vi "Config-Stress-Definition.vi"(6 "delete all units":bool, 8 "error in (no error)":errorcluster, 9 "comments (max 58 chars)":string, 10 "trigger (disable:0)":u16(ring), 11 "VISA session":refnum<visa-resource-name>) -> (0 "error out":errorcluster, 3 "VISA resource name out":refnum<visa-resource-name>)   [LabVIEW 2016, in "Agilent 415X Series.lvlib"]
doc: "This VI configures stress setting shared by all units (on stress group level)."
uses:
  Agilent 415X Series.lvlib
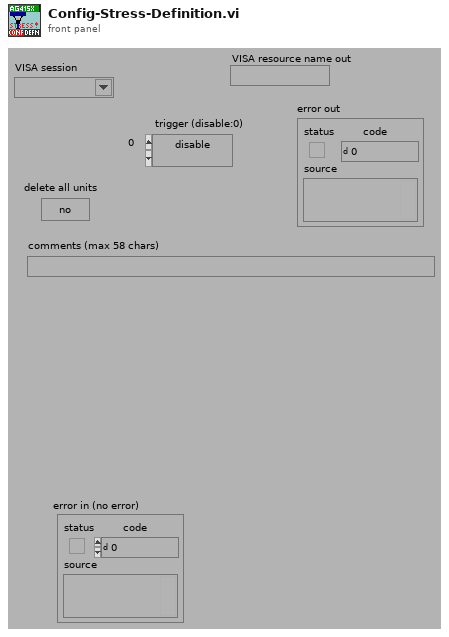
[diagram p1: front panel]
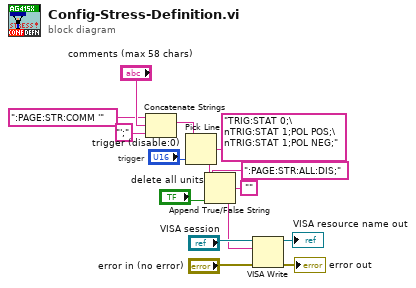
[diagram p0: block diagram]
diagram:
  # "trigger"
  n1 = Concatenate Strings(":PAGE:STR:COMM '", "comments (max 58 chars)", "';") -> (w11:string)
  n2 = Pick Line(string ("")=w11, multi-line string="TRIG:STAT 0;\nTRIG:STAT 1;POL POS;\nTRIG:STAT 1;POL NEG;", line index="trigger (disable:0)") -> (output string=w8:string)
  n3 = Append True/False String(1:"delete all units", 2:"", 3:":PAGE:STR:ALL:DIS;", 4:w8) -> (0:w2:string)
  n4 = VISA Write(VISA resource name="VISA session", write buffer=w2, error in (no error)="error in (no error)") -> (VISA resource name out=→"VISA resource name out":refnum<visa-resource-name>, error out=→"error out":errorcluster)  [unwired: 1 out]
